vi "Atto DRY Interface set Reservoir Tset Cold Sample.vi"(8 "error in (no error)":errorcluster, 11 "SetReservoirTsetColdSampleK":sgl) -> (0 "error out":errorcluster, 3 "function return":i32)   [LabVIEW 2016, in "attoDRYLib.lvlib"]
doc: "int32_t __cdecl AttoDRY_Interface_setReservoirTsetColdSample(\n float SetReservoirTsetColdSampleK);"
uses:
  <userlib>/attoDRYLib/attoDRYLib.lvlib
  <userlib>/attoDRYLib/attoDRYLib.dll
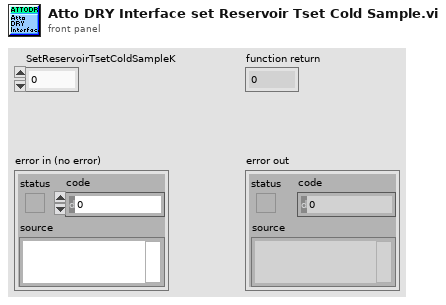
[diagram p1: front panel]
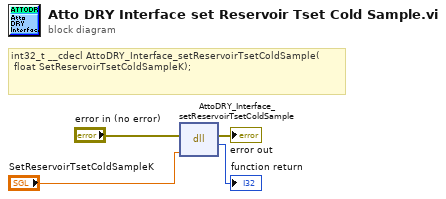
[diagram p0: block diagram]
diagram:
  # "int32_t __cdecl AttoDRY_Interface_setReservoirTsetColdSample(\n\tfloat SetReservoirTsetColdSampleK);"
  n1 = dll-call lib="C:/Program Files (x86)/National Instruments/LabVIEW 2016/user.lib/attoDRYLib/attoDRYLib.*" fn="AttoDRY_Interface_setReservoirTsetColdSample"(error in="error in (no error)", "SetReservoirTsetColdSampleK"="SetReservoirTsetColdSampleK") -> (error out=→"error out":errorcluster, →"function return":i32)  [unwired: 3 in, 1 out]
